vi "test_RPLiDAR_Main4.vi"() -> ()   [LabVIEW 2019]
uses:
  Ctrl/rplidar_cmd.ctl
panel:
  out "distance":dbl[](array[numeric])
  in  "Tab Control":enum32{"UI", "ref"}(tab)
  out "XY Graph 4":cluster{"X":dbl, "Y":dbl}[](graph)=[{"X"=0.015325048178804875, "Y"=-0.3283926086231499}, {"X"=0.011435999065957792, "Y"=-0.33805662310530676}, {"X"=0.006759964923129894, "Y"=-0.3349317883901706}, {"X"=0.0025998998912820153, "Y"=-0.3287397192621472}, {"X"=-0.0018497661882666344, "Y"=-0.3229947033080399}, {"X"=-0.015743555479908303, "Y"=-0.3496457356537486}]
  in  "speed":u16(slide)=272 scale=100.0..1000.0
  out "buffer":u32(graph)
  in  "Reset":bool
  in  "stop":bool
  out "dt_check":u32=20
  out "rs232 data":string
  in  "dt":u32=6
  out "response check":bool=TRUE
  out "n_enq":i32=7317
  out "n q buf":i32
  in  "Reset data":bool=TRUE
  out "real packet":bool
  in  "scan":bool
  in  "health":bool
  in  "stop":bool
  in  "spin":bool
  out "health check":bool=TRUE
  in  "close":bool
  out "XY Graph 3":cluster{"X":dbl, "Y":dbl}[](graph)=[{"X"=0.015325048178804875, "Y"=-0.3283926086231499}, {"X"=0.011435999065957792, "Y"=-0.33805662310530676}, {"X"=0.006759964923129894, "Y"=-0.3349317883901706}, {"X"=0.0025998998912820153, "Y"=-0.3287397192621472}, {"X"=-0.0018497661882666344, "Y"=-0.3229947033080399}, {"X"=-0.015743555479908303, "Y"=-0.3496457356537486}]
  out "read buffer":string
  out "update bit":bool
  in  "update n":u8=20
  out "error out":errorcluster
  in  "VLP16 cfg":T1={"h range"={82, -88}, "v range"={7, -9}} {"v range" scale=-15.0..15.0; "h range" scale=-180.0..180.0}
  in  "RPLidar cfg":T2={"port"="COM6", "dt"=6, "update n"=8, "speed"=272, "rate "=256000} {"speed" scale=100.0..1000.0}
  out "distance graph":dbl[](graph)
  out "angle graph":dbl[](graph)
  out "while loop n":i32
  out "for loop n":i32
  in  "인덱스":i32
  in  "길이":i32
  # "RPLIDAR"
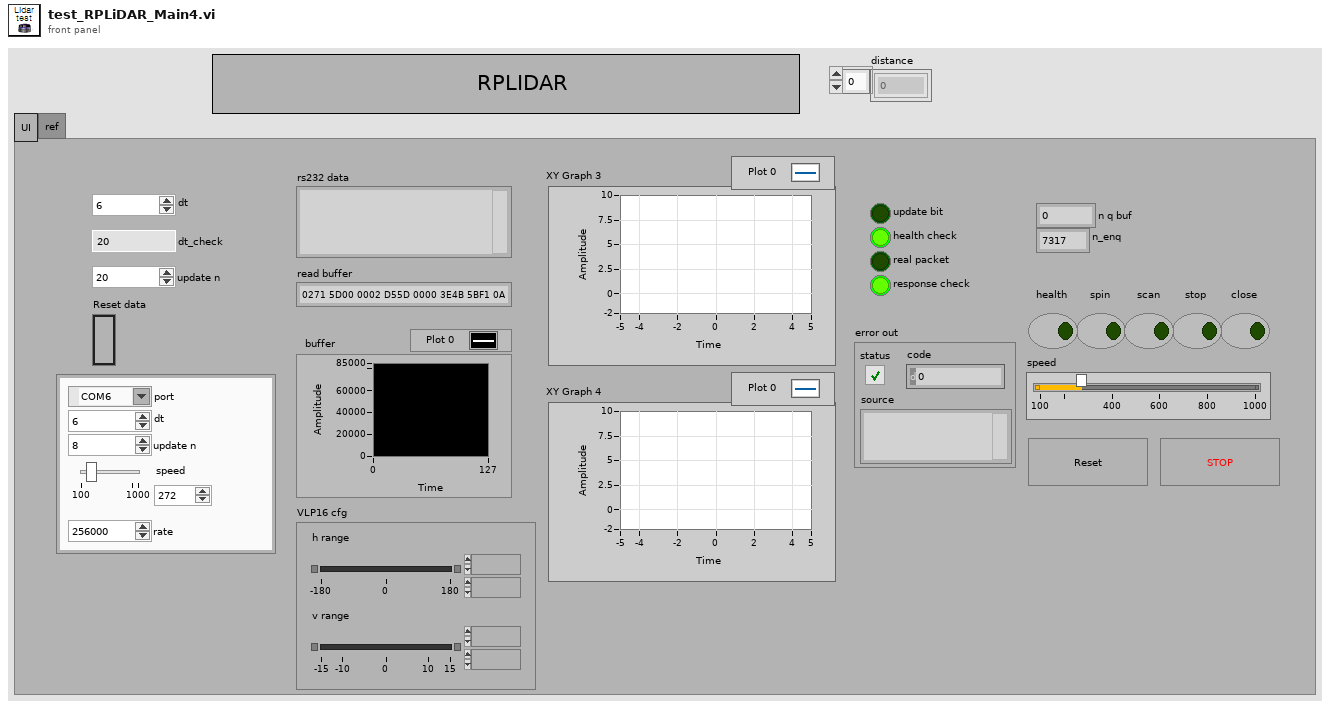
[diagram p1: front panel]
types:
  T1 = cluster{"h range":cluster{i16, i16}, "v range":cluster{i8, i8}}
  T2 = cluster{"port":refnum<visa-resource-name>, "dt":u32, "update n":u8, "speed":u16, "rate ":u32}
  T3 = typedef "rplidar_cmd.ctl" = enum16{"init", "health", "spin", "scan", "read", "stop", "close"}
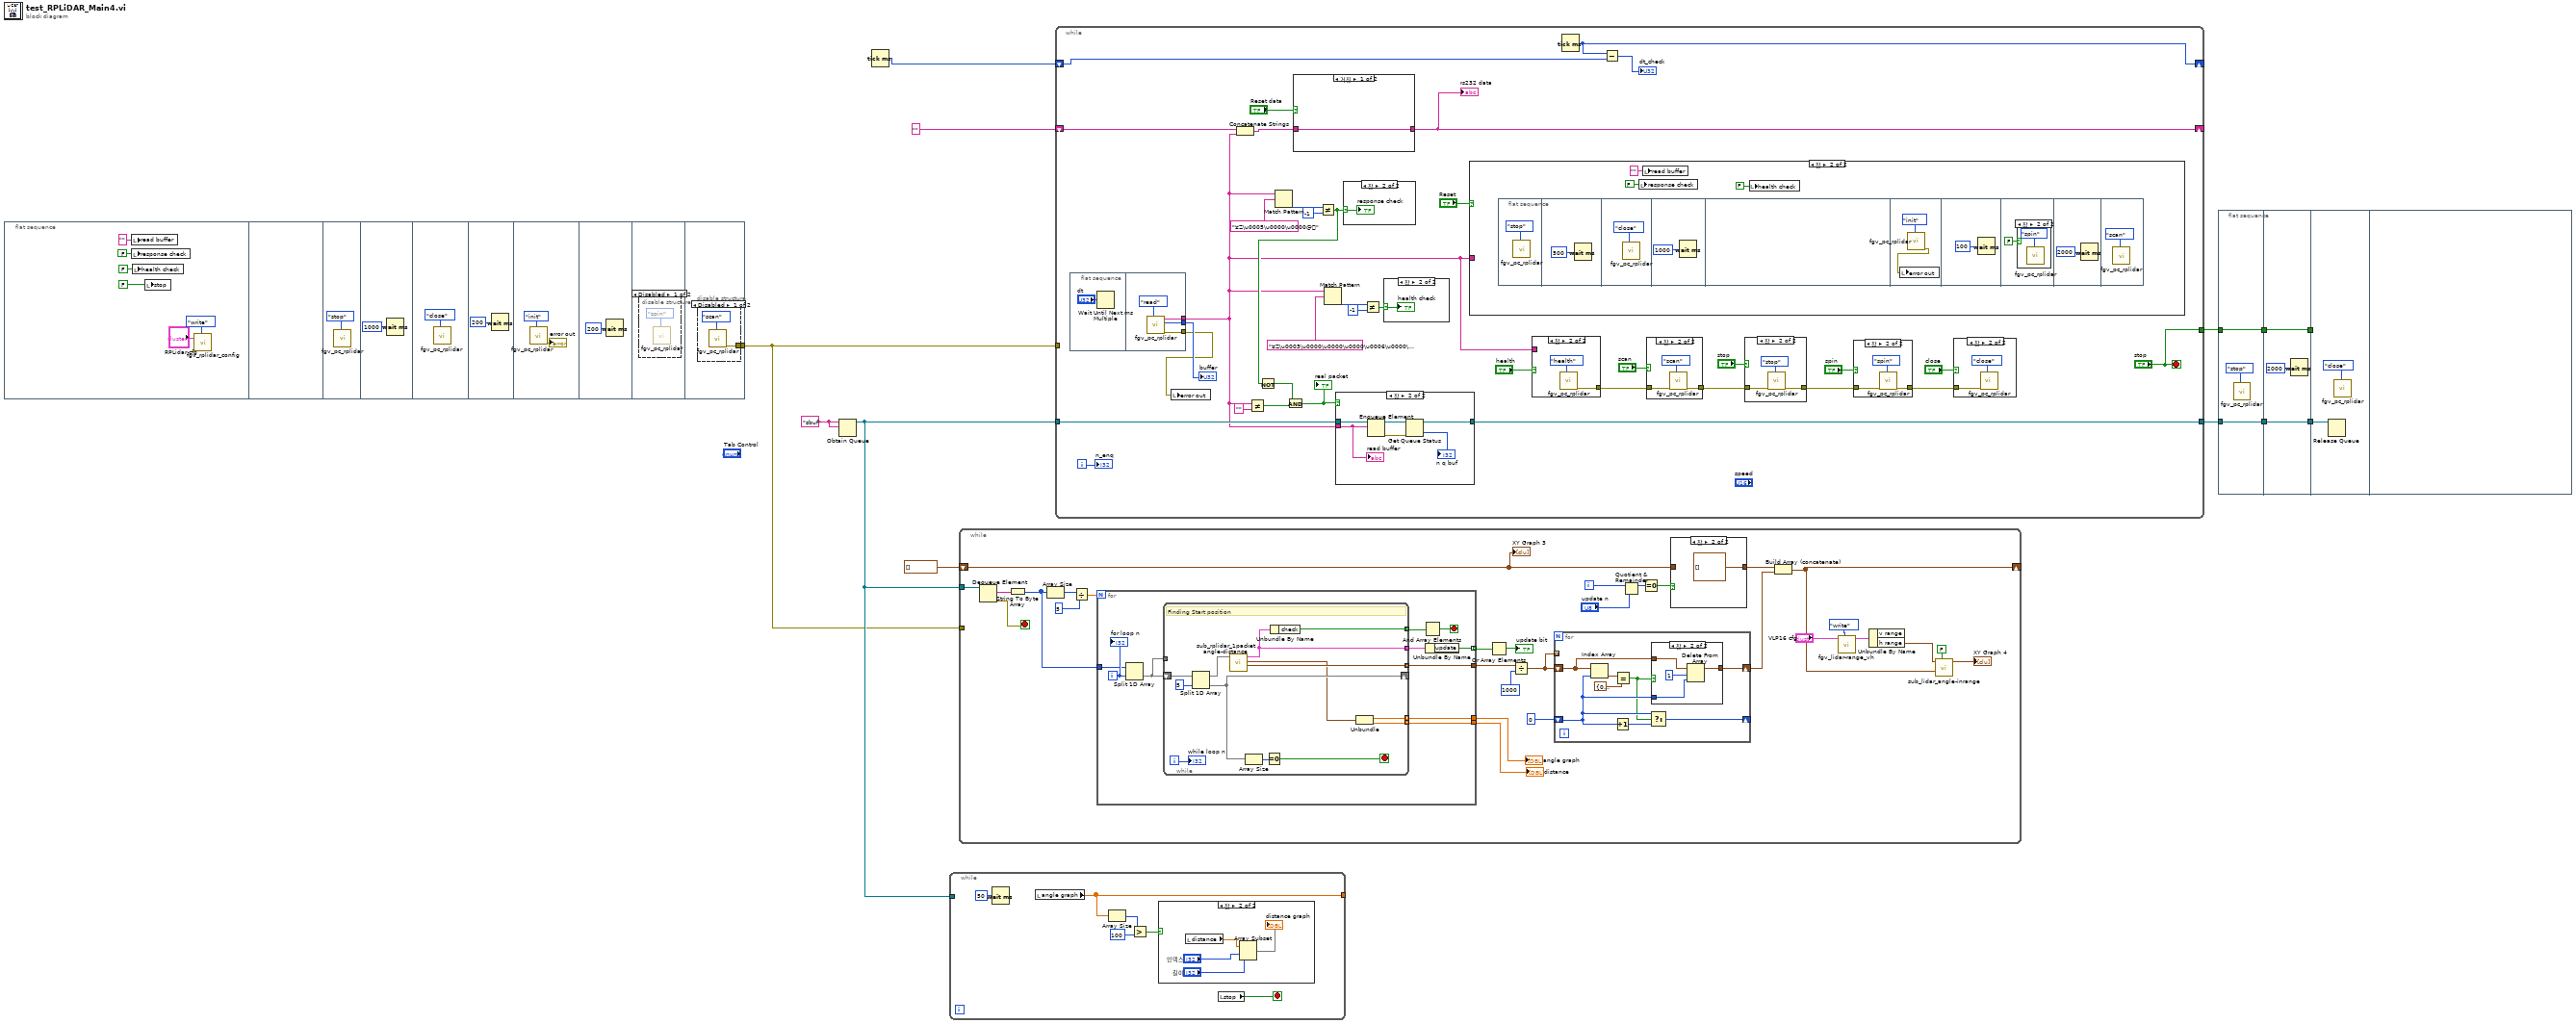
[diagram p0: block diagram]
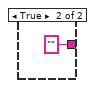
[diagram p13: hidden frame]
diagram:
  w10 = "sbuf" ("name (unnamed)")
  n1 = flat-sequence {
    tunnel: [w27] -> w1
    frame #0 {
      n2 = local write "read buffer"("" ("read buffer")) -> ()
      n3 = local write "response check"(FALSE ("response check")) -> ()
      n4 = local write "health check"(FALSE ("health check")) -> ()
      n5 = local write "stop"(FALSE ("health check")) -> ()
      n6 = call "fgv_rplidar_config.vi"("cmd"=enum16{"read", "write"}."write", "RPLidar cfg"="RPLidar cfg") -> ()  [unwired: 8 in, 2 out]
    }
    frame #1 {
    }
    frame #2 {
      n7 = call "fgv_pc_rplidar.vi"("cmd"=rplidar_cmd."stop") -> ()  [unwired: 8 in, 3 out]
    }
    frame #3 {
      n8 = Wait (ms)(milliseconds to wait=u32 1000) -> ()  [unwired: 1 out]
    }
    frame #4 {
      n9 = call "fgv_pc_rplidar.vi"("cmd"=rplidar_cmd."close") -> ()  [unwired: 8 in, 3 out]
    }
    frame #5 {
      n10 = Wait (ms)(milliseconds to wait=u32 200) -> ()  [unwired: 1 out]
    }
    frame #6 {
      n11 = call "fgv_pc_rplidar.vi"("cmd"=rplidar_cmd."init") -> ("error out"=→"error out":errorcluster)  [unwired: 8 in, 2 out]
    }
    frame #7 {
      n12 = Wait (ms)(milliseconds to wait=u32 200) -> ()  [unwired: 1 out]
    }
    frame #8 {
      n13 = disable-structure shown="Disabled" {
        frame Disabled {
          n14 = call "fgv_pc_rplidar.vi"("cmd"=rplidar_cmd."spin") -> ()  [unwired: 8 in, 3 out]
        }
        frame Enabled {
        }
      }
    }
    frame #9 {
      n15 = disable-structure shown="Disabled" {
        disable-tunnel: [w28 _] -> w27
        frame Disabled {
          n16 = call "fgv_pc_rplidar.vi"("cmd"=rplidar_cmd."scan") -> ("error out"=w28:errorcluster)  [unwired: 8 in, 2 out]
        }
        frame Enabled {
        }
      }
    }
  }
  n17 = Obtain Queue(name (unnamed)=w10, element data type=w10) -> (queue out=w2:refnum<queue>)  [unwired: 3 in, 2 out]
  n18 = Tick Count (ms)() -> (millisecond timer value=w11:u32)
  n19 = while {
    tunnel: w2 -> [_]
    tunnel: [w33] -> _
    stop <- w35 stop-if-true
    n20 = Wait (ms)(milliseconds to wait=u32 50 ("대기 시간 (ms)")) -> ()  [unwired: 1 out]
    n21 = local read "angle graph"() -> (w33:dbl[])
    n22 = Array Size(array=w33) -> (size(s)=w32:i32)
    n23 = Greater?(x=w32, y=100) -> (0:w30:bool)
    n24 = case shown="참" w30 {
      frame False {
      }
      frame True {
        n25 = local read "distance"() -> (w39:dbl[])
        n26 = Array Subset(array=w39, index="인덱스", length="길이") -> (→"distance graph":dbl[])
      }
    }
    n27 = local read "stop"() -> (w35:bool)
  }
  n28 = while {
    tunnel: w2 -> [w68]
    shift-right: [w43] -> _
    shift-left: cluster{dbl, dbl}[] [] -> [w49]
    tunnel: w1 -> [_]
    i -> [w54]
    stop <- w67 stop-if-true
    n29 = Dequeue Element(queue=w68) -> (element=w66:string, error out=w67:errorcluster)  [unwired: 2 in, 2 out]
    n30 = String To Byte Array(string=w66) -> (unsigned byte array=w65:u8[])
    n31 = Array Size(array=w65) -> (size(s)=w64:i32)
    n32 = Divide(x=w64, y=5) -> (x/y=w62:dbl)
    n33 = for {
      N: w62 -> [_]
      tunnel: w65 -> [w91]
      tunnel: [w86] -> w61
      tunnel: [w88] -> w55 mode=indexing
      tunnel: [w85] -> w48
      tunnel: [w84] -> w47
      i -> [w92]
      stop <- w93 stop-if-true
      n34 = Split 1D Array(array=w91, index=w92) -> (second subarray=w90:u8[])  [unwired: 1 out]
      n35 = while {
        tunnel: w90 -> [_]
        shift-right: [w105] -> _
        shift-left: w90 -> [w106]
        tunnel: [w97] -> w86 mode=indexing
        tunnel: [w100] -> w89
        tunnel: [w99] -> w87 mode=indexing
        tunnel: [w95] -> w85 mode=indexing
        tunnel: [w94] -> w84 mode=indexing
        i -> [w98]
        stop <- w103 stop-if-true
        # "Finding Start position"
        n36 = Split 1D Array(array=w106, index=5) -> (first subarray=w102:u8[], second subarray=w105:u8[])
        n37 = call "sub_rplidar_1packet angle-distance.vi"("packet"=w102) -> ("xy"=w97:cluster{"x":dbl, "y":dbl}, "angle distance"=w96:cluster{"angle":dbl, "distance":dbl}, "udate check"=w100:cluster{"update":bool, "check":bool})  [unwired: 8 in]
        n38 = Array Size(array=w105) -> (size(s)=w104:i32)
        n39 = Equal To 0?(x=w104) -> (x = 0?=w103:bool)
        n40 = Unbundle By Name(w100) -> ("check"=w99:bool)
        n41 = Unbundle(w96) -> ("angle"=w95:dbl, "distance"=w94:dbl)
        "while loop n" <- w98
      }
      n42 = And Array Elements(Boolean array=w87) -> (logical AND=w93:bool)
      n43 = Unbundle By Name(w89) -> ("update"=w88:bool)
      "for loop n" <- w92
    }
    "angle graph" <- w48
    "distance" <- w47
    n44 = Or Array Elements(Boolean array=w55) -> (logical OR=→"update bit":bool)
    n45 = Divide(x=w61, y=1000) -> (x/y=w58:cluster{"x":dbl, "y":dbl}[])
    n46 = for {
      tunnel: w58 -> [_] mode=indexing
      shift-right: [w75] -> w57
      shift-left: w58 -> [w71]
      shift-right: [w74] -> _
      shift-left: 0 -> [w73]
      n47 = Index Array(array=w71, index=w73) -> (element=w78:cluster{"x":dbl, "y":dbl})
      n48 = Increment(x=w73) -> (x+1=w76:i32)
      n49 = Equal?(x=w78, y=cluster{dbl, dbl} {0.0, -0.0}) -> (x = y?=w72:bool)
      n50 = Select(t=w73, s=w72, f=w76) -> (s? t:f=w74:i32)
      n51 = case shown="참" w72 {
        tunnel: w71 -> [w79 w83]
        tunnel: [w79 w82] -> w75
        tunnel: w73 -> [_ w80]
        frame False {
        }
        frame True {
          n52 = Delete From Array(array=w83, length=1, index=w80) -> (array with subset deleted=w82:cluster{"x":dbl, "y":dbl}[])  [unwired: 1 out]
        }
      }
    }
    n53 = Quotient & Remainder(x=w54, y="update n") -> (x-y*floor(x/y)=w53:i32)  [unwired: 1 out]
    n54 = Equal To 0?(x=w53) -> (x = 0?=w52:bool)
    n55 = case shown="참" w52 {
      tunnel: w49 -> [w69 _]
      tunnel: [w69 cluster{dbl, dbl}[] []] -> w56
      frame False {
      }
      frame True {
      }
    }
    n56 = Build Array (concatenate)(w56, w57) -> (w43:cluster{"x":dbl, "y":dbl}[])
    n57 = call "fgv_lidar-range_vh.vi"("cmd"=enum16{"read", "write"}."write", "VLP16 cfg"="VLP16 cfg") -> ("VLP16 cfg out"=w45:T1)  [unwired: 9 in]
    n58 = Unbundle By Name(w45) -> ("h range"=w41:cluster{i16, i16})  [unwired: 1 out]
    n59 = call "sub_lidar_angle-inrange.vi"("3d"=FALSE, "2D data"=w43, "h range"=w41) -> ("Array out"=→"XY Graph 4":cluster{"x":dbl, "y":dbl}[])  [unwired: 6 in, 2 out]
    "XY Graph 3" <- w49
  }
  n60 = while {
    tunnel: ["stop"] -> w12
    tunnel: w1 -> [_]
    shift-right: [w107] -> _
    shift-left: w11 -> [w139]
    shift-right: [w127] -> _
    shift-left: "" -> [w138]
    tunnel: w2 -> [w132]
    tunnel: [w131] -> w9
    i -> [w130]
    stop <- "stop" stop-if-true
    n61 = flat-sequence {
      tunnel: [w188] -> w113
      tunnel: [w186] -> w140
      tunnel: [w185] -> w108
      frame #0 {
        n62 = Wait Until Next ms Multiple(millisecond multiple="dt") -> ()  [unwired: 1 out]
      }
      frame #1 {
        n63 = call "fgv_pc_rplidar.vi"("cmd"=rplidar_cmd."read") -> ("error out"=w185:errorcluster, "serial buf"=w186:u32, "read buffer"=w188:string)  [unwired: 8 in]
      }
    }
    n64 = local write "error out"(w108) -> ()
    n65 = Concatenate Strings(w138, w113) -> (w137:string)
    n66 = Not Equal?(x=w113, y="") -> (x != y?=w126:bool)
    n67 = Match Pattern(string=w113, regular expression="¥Z\u0005\u0000\u0000@") -> (offset past match=w135:i32)  [unwired: 1 in, 3 out]
    n68 = case shown="거짓" "Reset data" {
      tunnel: w137 -> [w160 _]
      tunnel: [w160 ""] -> w127
      frame False {
      }
      frame True {
      }
    }
    "rs232 data" <- w127
    n69 = Not Equal?(x=w135, y=-1) -> (x != y?=w125:bool)
    n70 = Not(x=w125) -> (.not. x?=w123:bool)
    n71 = And(x=w123, y=w126) -> (x .and. y?=w124:bool)
    "real packet" <- w124
    n72 = Match Pattern(string=w113, regular expression="¥Z\u0003\u0000\u0000\u0000\u0006\u0000\u0000\u0000") -> (offset past match=w115:i32)  [unwired: 1 in, 3 out]
    n73 = case shown="참" w124 {
      tunnel: w132 -> [w162 w168]
      tunnel: [w162 w165] -> w131
      tunnel: w113 -> [_ w163]
      frame False {
      }
      frame True {
        n74 = Enqueue Element(queue=w168, element=w163) -> (queue out=w167:refnum<queue>, error out=w164:errorcluster)  [unwired: 2 in, 1 out]
        n75 = Get Queue Status(queue=w167, error in (no error)=w164) -> (queue out=w165:refnum<queue>, # elements in queue=→"n q buf":i32)  [unwired: 1 in, 6 out]
        "read buffer" <- w163
      }
    }
    n76 = case shown="참" w125 {
      selector: w125 -> [_ w183]
      frame False {
      }
      frame True {
        "response check" <- w183
      }
    }
    n77 = Not Equal?(x=w115, y=-1) -> (x != y?=w117:bool)
    n78 = case shown="참" w117 {
      selector: w117 -> [_ w143]
      frame False {
      }
      frame True {
        "health check" <- w143
      }
    }
    n79 = case shown="참" "Reset" {
      tunnel: w113 -> [_ _]
      frame False {
      }
      frame True {
        n80 = flat-sequence {
          frame #0 {
            n81 = call "fgv_pc_rplidar.vi"("cmd"=rplidar_cmd."stop") -> ()  [unwired: 8 in, 3 out]
          }
          frame #1 {
            n82 = Wait (ms)(milliseconds to wait=u32 500) -> ()  [unwired: 1 out]
          }
          frame #2 {
            n83 = call "fgv_pc_rplidar.vi"("cmd"=rplidar_cmd."close") -> ()  [unwired: 8 in, 3 out]
          }
          frame #3 {
            n84 = Wait (ms)(milliseconds to wait=u32 1000) -> ()  [unwired: 1 out]
          }
          frame #4 {
          }
          frame #5 {
            n85 = call "fgv_pc_rplidar.vi"("cmd"=rplidar_cmd."init") -> ("error out"=w176:errorcluster)  [unwired: 8 in, 2 out]
            n86 = local write "error out"(w176) -> ()
          }
          frame #6 {
            n87 = Wait (ms)(milliseconds to wait=u32 100) -> ()  [unwired: 1 out]
          }
          frame #7 {
            n88 = case shown="참" FALSE {
              frame False {
              }
              frame True {
                n89 = call "fgv_pc_rplidar.vi"("cmd"=rplidar_cmd."spin") -> ()  [unwired: 8 in, 3 out]
              }
            }
          }
          frame #8 {
            n90 = Wait (ms)(milliseconds to wait=u32 2000) -> ()  [unwired: 1 out]
          }
          frame #9 {
            n91 = call "fgv_pc_rplidar.vi"("cmd"=rplidar_cmd."scan") -> ()  [unwired: 8 in, 3 out]
          }
        }
        n92 = local write "response check"(FALSE ("response check")) -> ()
        n93 = local write "read buffer"("" ("read buffer")) -> ()
        n94 = local write "health check"(FALSE ("health check")) -> ()
      }
    }
    n95 = case shown="참" "health" {
      tunnel: w113 -> [_ _]
      tunnel: [_ w158] -> w112
      frame False {
      }
      frame True {
        n96 = call "fgv_pc_rplidar.vi"("cmd"=rplidar_cmd."health") -> ("error out"=w158:errorcluster)  [unwired: 8 in, 2 out]
      }
    }
    n97 = Tick Count (ms)() -> (millisecond timer value=w107:u32)
    n98 = Subtract(x=w107, y=w139) -> (x-y=→"dt_check":u32)
    n99 = case shown="참" "scan" {
      tunnel: w112 -> [w154 w156]
      tunnel: [w154 w155] -> w111
      frame False {
      }
      frame True {
        n100 = call "fgv_pc_rplidar.vi"("cmd"=rplidar_cmd."scan", "error in"=w156) -> ("error out"=w155:errorcluster)  [unwired: 7 in, 2 out]
      }
    }
    n101 = case shown="참" "stop" {
      tunnel: w111 -> [w150 w152]
      tunnel: [w150 w151] -> w110
      frame False {
      }
      frame True {
        n102 = call "fgv_pc_rplidar.vi"("cmd"=rplidar_cmd."stop", "error in"=w152) -> ("error out"=w151:errorcluster)  [unwired: 7 in, 2 out]
      }
    }
    n103 = case shown="참" "spin" {
      tunnel: w110 -> [w146 w148]
      tunnel: [w146 w147] -> w109
      frame False {
      }
      frame True {
        n104 = call "fgv_pc_rplidar.vi"("cmd"=rplidar_cmd."spin", "error in"=w148) -> ("error out"=w147:errorcluster)  [unwired: 7 in, 2 out]
      }
    }
    n105 = case shown="참" "close" {
      tunnel: w109 -> [_ w144]
      frame False {
      }
      frame True {
        n106 = call "fgv_pc_rplidar.vi"("cmd"=rplidar_cmd."close", "error in"=w144) -> ()  [unwired: 7 in, 3 out]
      }
    }
    "buffer" <- w140
    "n_enq" <- w130
  }
  n107 = flat-sequence {
    tunnel: w9 -> [w190]
    tunnel: w12 -> [w191]
    tunnel: [w191] -> w6
    tunnel: [w190] -> w4
    tunnel: w6 -> [w194]
    tunnel: [w194] -> w5
    tunnel: w4 -> [w193]
    tunnel: [w193] -> w3
    tunnel: w5 -> [_]
    tunnel: w3 -> [w195]
    frame #0 {
      n108 = call "fgv_pc_rplidar.vi"("cmd"=rplidar_cmd."stop") -> ()  [unwired: 8 in, 3 out]
    }
    frame #1 {
      n109 = Wait (ms)(milliseconds to wait=u32 2000) -> ()  [unwired: 1 out]
    }
    frame #2 {
      n110 = Release Queue(queue=w195) -> ()  [unwired: 2 in, 3 out]
      n111 = call "fgv_pc_rplidar.vi"("cmd"=rplidar_cmd."close") -> ()  [unwired: 8 in, 3 out]
    }
    frame #3 {
    }
  }
